vi "mqttCmdSubscribeSubInfoRead.vi"(0 "mqttSubscribe in":refnum<class "mqttCmdSubscribe.lvclass">, 11 "error in (no error)":errorcluster) -> (4 "mqttSubscribe out":refnum<class "mqttCmdSubscribe.lvclass">, 6 "subscriptionInfo":T1[](array[typedef])=[{"Topic"="a/b", "QoS"=enum."At least once"}], 15 "error out":errorcluster)   [LabVIEW 2020, in "mqttCmdSubscribe.lvclass"]
uses:
  mqttCmdSubscribe.lvclass
  mqttTypedef/mqttSubscribeCluster.ctl
  mqttTypedef/mqttQOSlevel.ctl
  mqttCmdSubscribe.lvclass/mqttCmdSubscribe.ctl
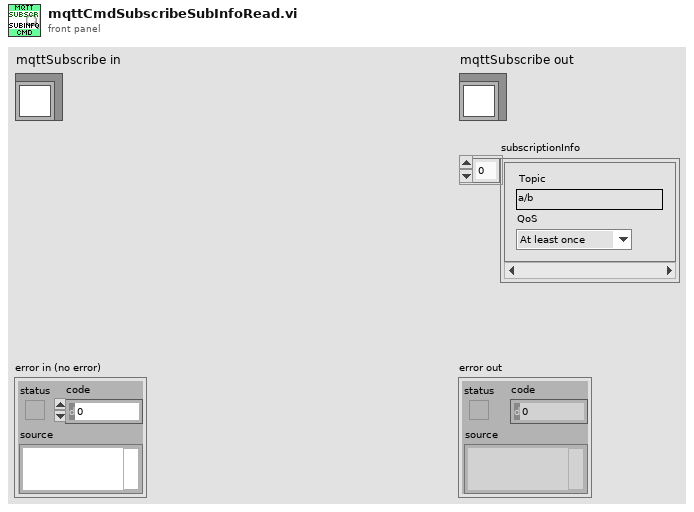
[diagram p1: front panel]
types:
  T1 = typedef "mqttSubscribeCluster.ctl" = cluster{"Topic":string, "QoS":T2}
  T2 = typedef "mqttQOSlevel.ctl" = enum8{"At most once", "At least once", "Exactly once", "Reserved"}
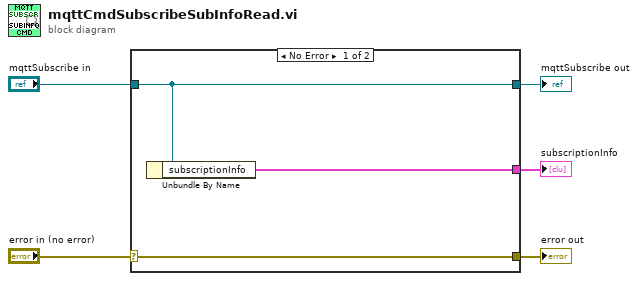
[diagram p0: block diagram]
diagram:
  n1 = case shown="No Error" "error in (no error)" {
    selector: "error in (no error)" -> [w8 w9]
    tunnel: [w8 w9] -> w4
    tunnel: [w7 w10] -> w2
    tunnel: "mqttSubscribe in" -> [w7 w10]
    tunnel: [w6 _] -> w1
    frame No Error {
      n2 = Unbundle By Name(w7) -> ("subscriptionInfo"=w6:T1[])
    }
    frame Error {
    }
  }
  "error out" <- w4
  "mqttSubscribe out" <- w2
  "subscriptionInfo" <- w1
